vi "Create Server Class from Template.vi"(7 "gRPC Method Parameters":T1[](array[typedef]), 8 "error in (no error)":errorcluster, 10 "Library":refnum<vi>, 11 "Application ref in":refnum<vi>) -> (0 "error out":errorcluster, 2 "Already Exists ?":bool, 3 "LVClassLibrary in":refnum<vi>)   [LabVIEW 2019, in "gRPC Template Creation Utility.lvlib"]
uses:
  gRPC Template Creation Utility.lvlib
  TypeDefs/RPC Method Parameters.ctl
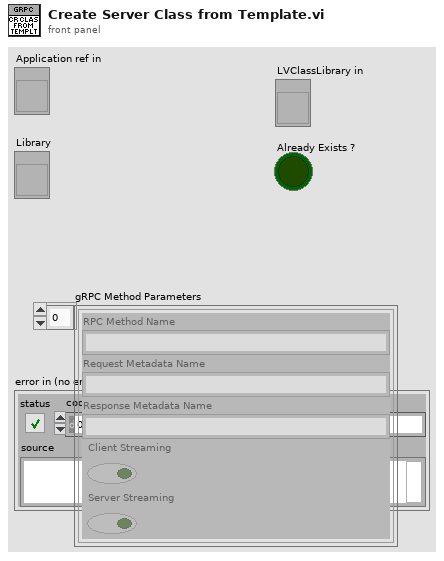
[diagram p1: front panel]
types:
  T1 = typedef "gRPC Template Creation Utility.lvlib/RPC Method Parameters.ctl" = cluster{"RPC Method Name":string, "Request Metadata Name":string, "Response Metadata Name":string, "Client Streaming":bool, "Server Streaming":bool}
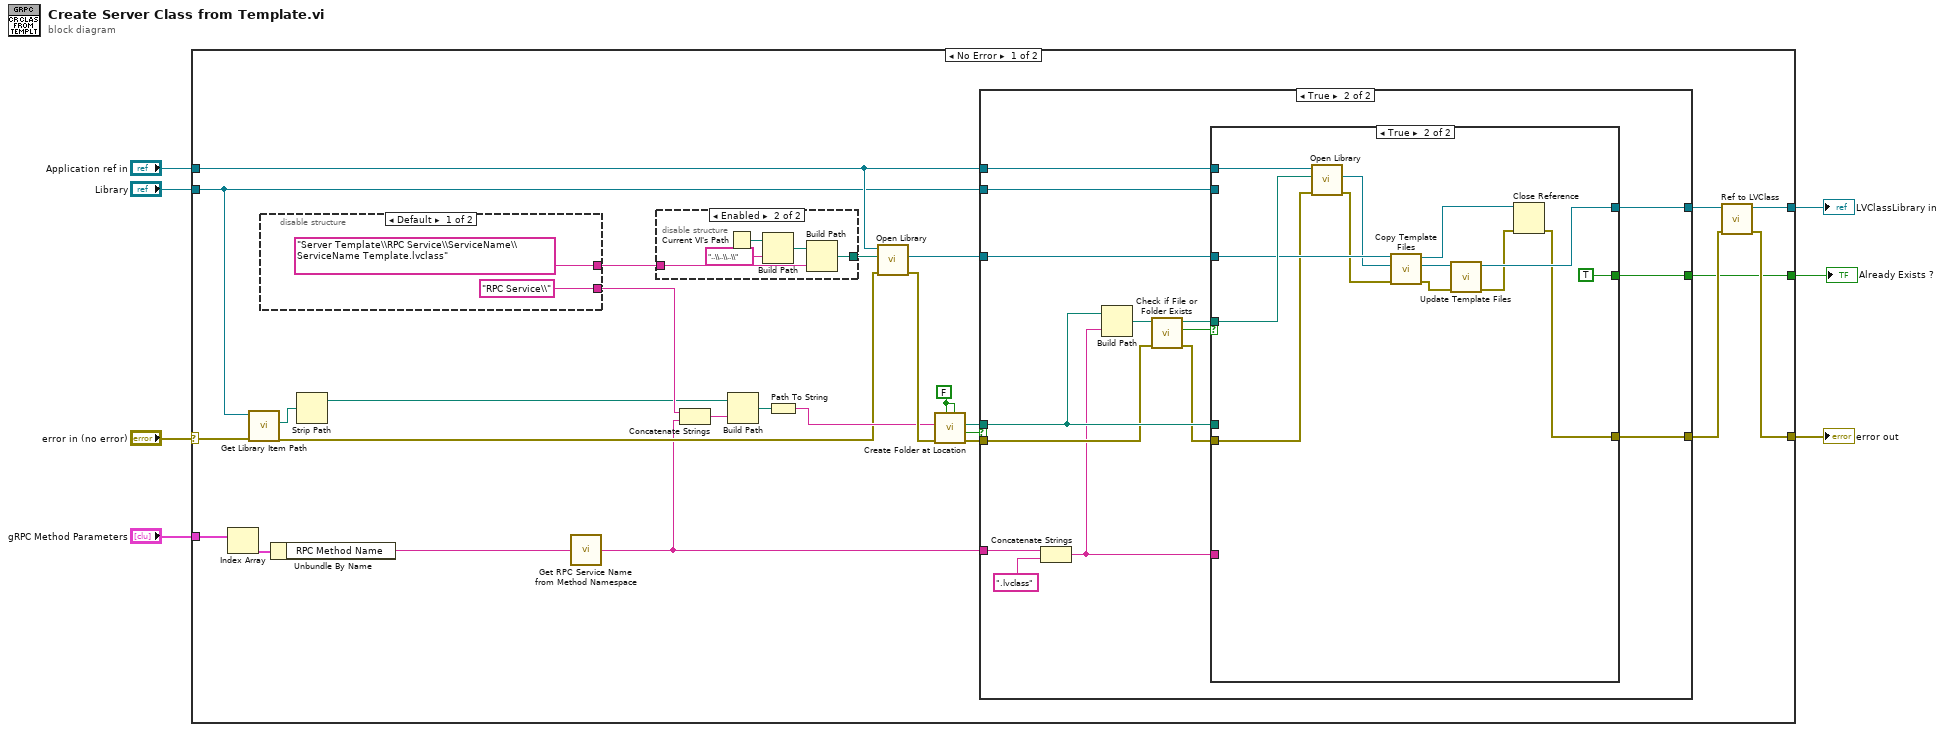
[diagram p0: block diagram]
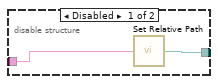
[diagram p2: hidden frame]
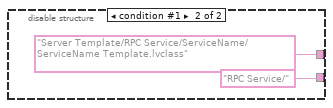
[diagram p3: hidden frame]
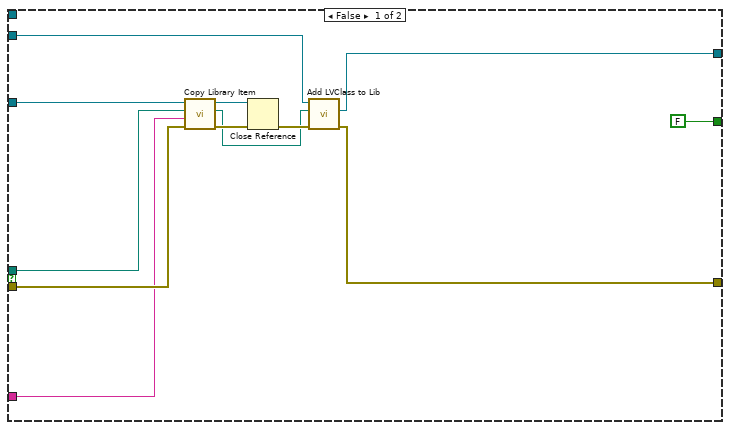
[diagram p4: hidden frame]
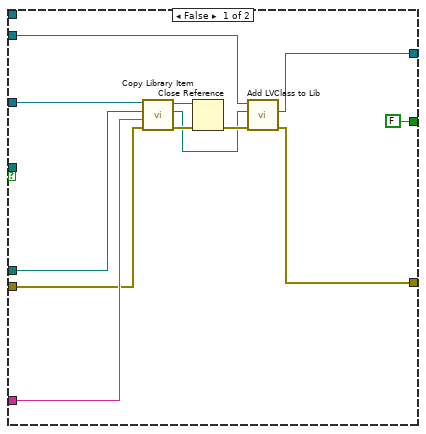
[diagram p5: hidden frame]
diagram:
  n1 = case shown="No Error" "error in (no error)" {
    selector: "error in (no error)" -> [w15 w98]
    tunnel: [w16 w98] -> w7
    tunnel: [w18 _] -> w6
    tunnel: "Application ref in" -> [w25 _]
    tunnel: "gRPC Method Parameters" -> [w21 _]
    tunnel: "Library" -> [w13 _]
    tunnel: [w10 _] -> w1
    frame No Error {
      w29 = FALSE ("Use Relative")
      n2 = Index Array(array=w21) -> (element=w20:T1)  [unwired: 1 in]
      n3 = call "Get Library Item Path.vi"("error in (no error)"=w15, "Library"=w13) -> ("error out"=w14:errorcluster, "Path"=w12:path)  [unwired: 7 in, 1 out]
      n4 = disable-structure shown="Default" {
        disable-tunnel: ["Server Template\\RPC Service\\ServiceName\\ServiceName Template.lvclass" ("Application Relative Path") "Server Template/RPC Service/ServiceName/ServiceName Template.lvclass" ("Application Relative Path")] -> w23
        disable-tunnel: ["RPC Service\\" ("Path") "RPC Service/" ("Path")] -> w22
        frame condition #0 (active) {
        }
        frame condition #1 {
        }
      }
      n5 = Unbundle By Name(w20) -> ("RPC Method Name"=w9:string)
      n6 = Strip Path(path=w12) -> (stripped path=w11:path)  [unwired: 1 out]
      n7 = call "Get RPC Service Name from Method Namespace.vi"("RPC Method Name"=w9) -> ("RPC Service Name"=w8:string)
      n8 = disable-structure shown="Enabled" {
        disable-tunnel: [w36 w39] -> w32
        disable-tunnel: w23 -> [w35 w37]
        frame Disabled {
          n9 = call "Set Relative Path.vi"("Application Relative Path"=w35) -> ("Full Path"=w36:path)
        }
        frame Enabled {
          n10 = Current VI's Path() -> (path=w41:path)
          n11 = Build Path(base path=w41, name or relative path="..\\..\\..\\") -> (appended path=w38:path)
          n12 = Build Path(base path=w38, name or relative path=w37) -> (appended path=w39:path)
        }
      }
      n13 = Concatenate Strings(w22, w8) -> (w28:string)
      n14 = Build Path(base path=w11, name or relative path=w28) -> (appended path=w27:path)
      n15 = Path To String(path=w27) -> (string=w26:string)
      n16 = call "Open Library.vi"("error in (no error)"=w14, "Full Path"=w32, "Application in"=w25) -> ("error out"=w33:errorcluster, "Library out"=w30:refnum<vi>)  [unwired: 6 in, 1 out]
      n17 = call "Create Folder at Location.vi"("Override existing (F)"=w29, "Use Relative (F)"=w29, "Error In"=w33, "Path"=w26) -> ("Error Out"=w34:errorcluster, "Already Exists ?"=w24:bool, "Full path out"=w31:path)  [unwired: 5 in]
      n18 = case shown="True" w24 {
        tunnel: [w50 w64] -> w17
        tunnel: [w47 w69] -> w19
        tunnel: w34 -> [w55 w62]
        tunnel: w31 -> [w54 w66]
        tunnel: w30 -> [w53 w67]
        tunnel: w8 -> [w52 w65]
        tunnel: w25 -> [_ w68]
        tunnel: w13 -> [w49 w59]
        tunnel: [FALSE w58] -> w10
        frame False {
          n19 = call "Copy Library Item.vi"("error in (no error)"=w55, "Copy Name"=w52, "Copy location"=w54, "Library in"=w53) -> ("error out"=w57:errorcluster, "New Lib Path"=w48:path, "Library out"=w56:refnum<vi>)  [unwired: 5 in]
          n20 = Close Reference(reference=w56, error in (no error)=w57) -> (error out=w51:errorcluster)
          n21 = call "Add LVClass to Lib.vi"("error in (no error)"=w51, "LVClass Path in"=w48, "Library in"=w49) -> ("error out"=w50:errorcluster, "LVClassLibrary out"=w47:refnum<vi>)  [unwired: 6 in, 1 out]
        }
        frame True {
          n22 = Concatenate Strings(w65, ".lvclass" ("string")) -> (w60:string)
          n23 = Build Path(base path=w66, name or relative path=w60) -> (appended path=w71:path)
          n24 = call <vilib>:"Check if File or Folder Exists.vi"("error in (no error)"=w62, "path"=w71) -> ("error out"=w61:errorcluster, "file or folder exists?"=w70:bool, "dup path"=w63:path)  [unwired: 7 in]
          n25 = case shown="True" w70 {
            tunnel: [w82 w96] -> w69
            tunnel: w68 -> [_ w97]
            tunnel: w67 -> [w81 w93]
            tunnel: w66 -> [w80 _]
            tunnel: w60 -> [w79 _]
            tunnel: w61 -> [w78 w92]
            tunnel: [w77 w95] -> w64
            tunnel: w63 -> [_ w94]
            tunnel: w59 -> [w75 _]
            tunnel: [FALSE TRUE] -> w58
            frame False {
              n26 = call "Copy Library Item.vi"("error in (no error)"=w78, "Copy Name"=w79, "Copy location"=w80, "Library in"=w81) -> ("error out"=w84:errorcluster, "New Lib Path"=w74:path, "Library out"=w83:refnum<vi>)  [unwired: 5 in]
              n27 = Close Reference(reference=w83, error in (no error)=w84) -> (error out=w76:errorcluster)
              n28 = call "Add LVClass to Lib.vi"("error in (no error)"=w76, "LVClass Path in"=w74, "Library in"=w75) -> ("error out"=w77:errorcluster, "LVClassLibrary out"=w82:refnum<vi>)  [unwired: 6 in, 1 out]
            }
            frame True {
              n29 = call "Open Library.vi"("error in (no error)"=w92, "Full Path"=w94, "Application in"=w97) -> ("error out"=w91:errorcluster, "Library out"=w88:refnum<vi>)  [unwired: 6 in, 1 out]
              n30 = call "Copy Template Files.vi"("error in (no error)"=w91, "Server Library (Library Item) in"=w88, "Template Library (Library Item) in"=w93) -> ("error out"=w87:errorcluster, "Server Library (Library Item) out"=w86:refnum<vi>, "Template Library (Library Item) out"=w89:refnum<vi>)  [unwired: 6 in]
              n31 = call "Update Template Files.vi"("error in (no error)"=w87, "Server Library (Library Item) in"=w86) -> ("error out"=w90:errorcluster, "Server Library (Library Item) out"=w96:refnum<vi>)  [unwired: 8 in]
              n32 = Close Reference(reference=w89, error in (no error)=w90) -> (error out=w95:errorcluster)
            }
          }
        }
      }
      n33 = call "Ref to LVClass.vi"("error in (no error)"=w17, "ProjectItem in"=w19) -> ("error out"=w16:errorcluster, "LVClassLibrary out"=w18:refnum<vi>)  [unwired: 8 in]
    }
    frame Error {
    }
  }
  "error out" <- w7
  "LVClassLibrary in" <- w6
  "Already Exists ?" <- w1
